vi "Goto.vi"(6 "Home?":bool, 7 "Speed":i32, 8 "error in (no error)":errorcluster, 9 "channel":i32(ring)=1 items=["Channel1"=1, "Channel2"=2, "Channel3"=3, "Channel4"=4], 10 "New Position":sgl, 11 "TranslationStage in":refnum<class "BPC30x.lvclass">) -> (0 "error out":errorcluster, 3 "TranslationStage out":refnum<class "BPC30x.lvclass">)   [LabVIEW 2023, in "BPC30x.lvlib" / "BPC30x.lvclass"]
uses:
  BPC30x.lvclass
  UIs/TranslationStage_UI/TranslationStage_UI/StageMoveDone_For_UI.ctl
  <vilib>/ActorFramework/Actor/Actor.lvclass/Actor.ctl
  BPC30x.lvclass/BPC30x.ctl
  Interfaces/AbstractInstrumentClasses/TranslationStages_LV/TranslationStagesComm Messages/StageMoveDone Msg/StageMoveDone Msg.lvclass/StageMoveDone Msg.ctl
  <vilib>/ActorFramework/Message Enqueuer/Message Enqueuer.lvclass/Message Enqueuer.ctl
  <vilib>/ActorFramework/Message Enqueuer/Enqueue.vi
  Interfaces/AbstractInstrumentClasses/TranslationStages_LV/TranslationStagesComm Messages/StageMoveDone Msg/StageMoveDone Msg.lvclass
  <vilib>/ActorFramework/Message Priority Queue/Priority Enqueue.vi
  C:/Users/quantum/Documents/LVDAQ/UIs/TranslationStage_UI/Thorlabs.MotionControl.Benchtop.PiezoCLI.dll
  UIs/TranslationStage_UI/Thorlabs.MotionControl.Benchtop.PiezoCLI.dll
  <vilib>/ActorFramework/Actor/Actor.lvclass
  typedefs/typedefs.lvlib
panel:
  in  "Positions":T1={"CH1 Pos"=0.0, "CH2 Pos"=0.0, "CH3 Pos"=0.0, "CH4 Pos"=0.0, "Home?"=TRUE}
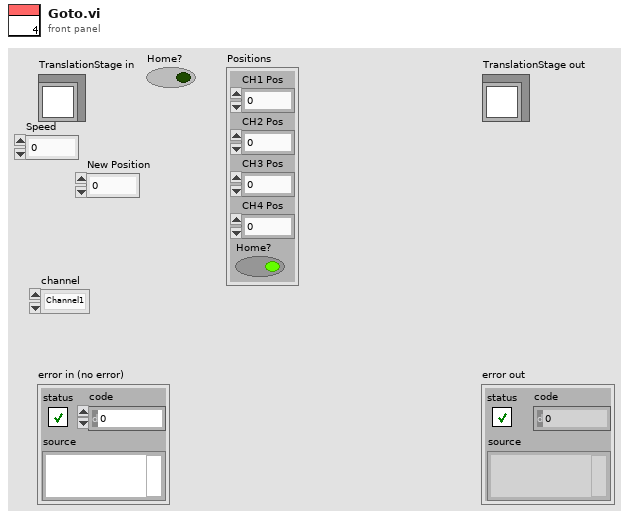
[diagram p1: front panel]
types:
  T1 = typedef "typedefs.lvlib/StageMoveDone_For_UI.ctl" = cluster{"CH1 Pos":sgl, "CH2 Pos":dbl, "CH3 Pos":dbl, "CH4 Pos":dbl, "Home?":bool}
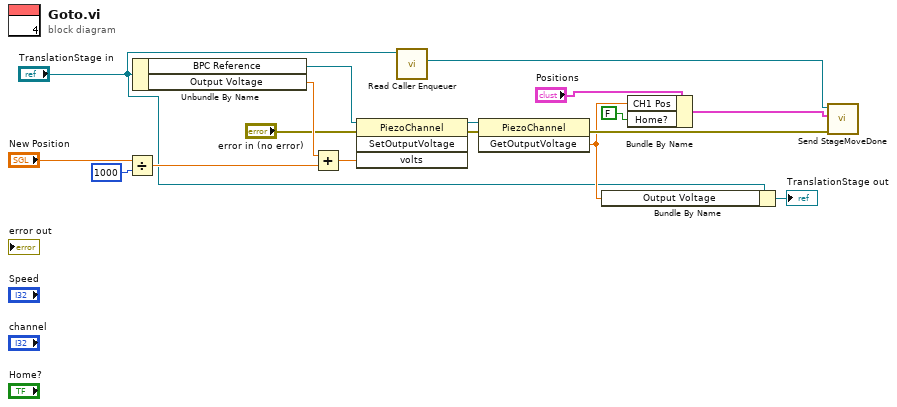
[diagram p0: block diagram]
diagram:
  n1 = Divide(x="New Position", y=u32 1000 ("x")) -> (x/y=w12:sgl)
  n2 = Unbundle By Name("TranslationStage in") -> ("BPC Reference"=w8:refnum<k24>, "Output Voltage"=w17:dbl)
  n3 = Add(x=w17, y=w12) -> (x+y=w16:dbl)
  n4 = invoke class="PiezoChannel" method="SetOutputVoltage"(reference=w8, error in="error in (no error)", "volts"=w16) -> (reference out=w11:refnum<k24>, error out=w10:errorcluster)  [unwired: 1 in, 2 out]
  n5 = call <vilib>:"Read Caller Enqueuer.vi"("Actor"="TranslationStage in") -> ("Caller Enqueuer"=w15:refnum<class "Message Enqueuer.lvclass">)  [unwired: 10 in]
  n6 = invoke class="PiezoChannel" method="GetOutputVoltage"(reference=w11, error in=w10) -> (error out=w9:errorcluster, "GetOutputVoltage"=w7:dbl)  [unwired: 1 in, 1 out]
  n7 = Bundle By Name(cluster="TranslationStage in", "Output Voltage"=w7) -> (→"TranslationStage out":refnum<class "BPC30x.lvclass">)
  n8 = Bundle By Name(cluster="Positions", "CH1 Pos"=w7, "Home?"=FALSE) -> (w3:T1)
  n9 = call "Send StageMoveDone.vi"("error in (no error)"=w9, "Positions"=w3, "Message Enqueuer"=w15) -> ()  [unwired: 7 in, 2 out]
